vi "Plot Sequence.vi"(5 "Strain Points":dbl[](array[numeric]), 6 "Sliders":T1 {"Instrument Sequence" scale=0.0..1.0; "Strain Sequence" scale=0.0..4.0}, 7 "Instrument Steps":T2, 8 "error in (no error)":errorcluster, 9 "Refnums":T10, 10 "Measurement":T5, 11 "Function":T9) -> (0 "error out":errorcluster)   [LabVIEW 2014]
uses:
  PlotData Refnums.ctl
  Chooseplot.ctl
  Electrical Data Plot Refnums.ctl
  Optical Spectrum Plot Refnum.ctl
  PlotData Functions.ctl
  Measurement.ctl
  WhichInstrument.ctl
  Hardware Control/Parameter Analyzer/Electrical Data.ctl
  Hardware Control/Spectrometer/Spectral Data.ctl
  Instrument Sequence/Instrument Steps.ctl
  Instrument Sequence/Action.ctl
  Instrument Sequence/Instrument List.ctl
panel:
  out "Configuration":string
  out "Measurement Sequence":cluster{"Instrument Sequence":T5[]}[](array[cluster])
  # "LICENSED MATERIALS – PROPERTY OF IBM\nCopyright IBM Corp. 2016,\nALL RIGHTS RESERVED"
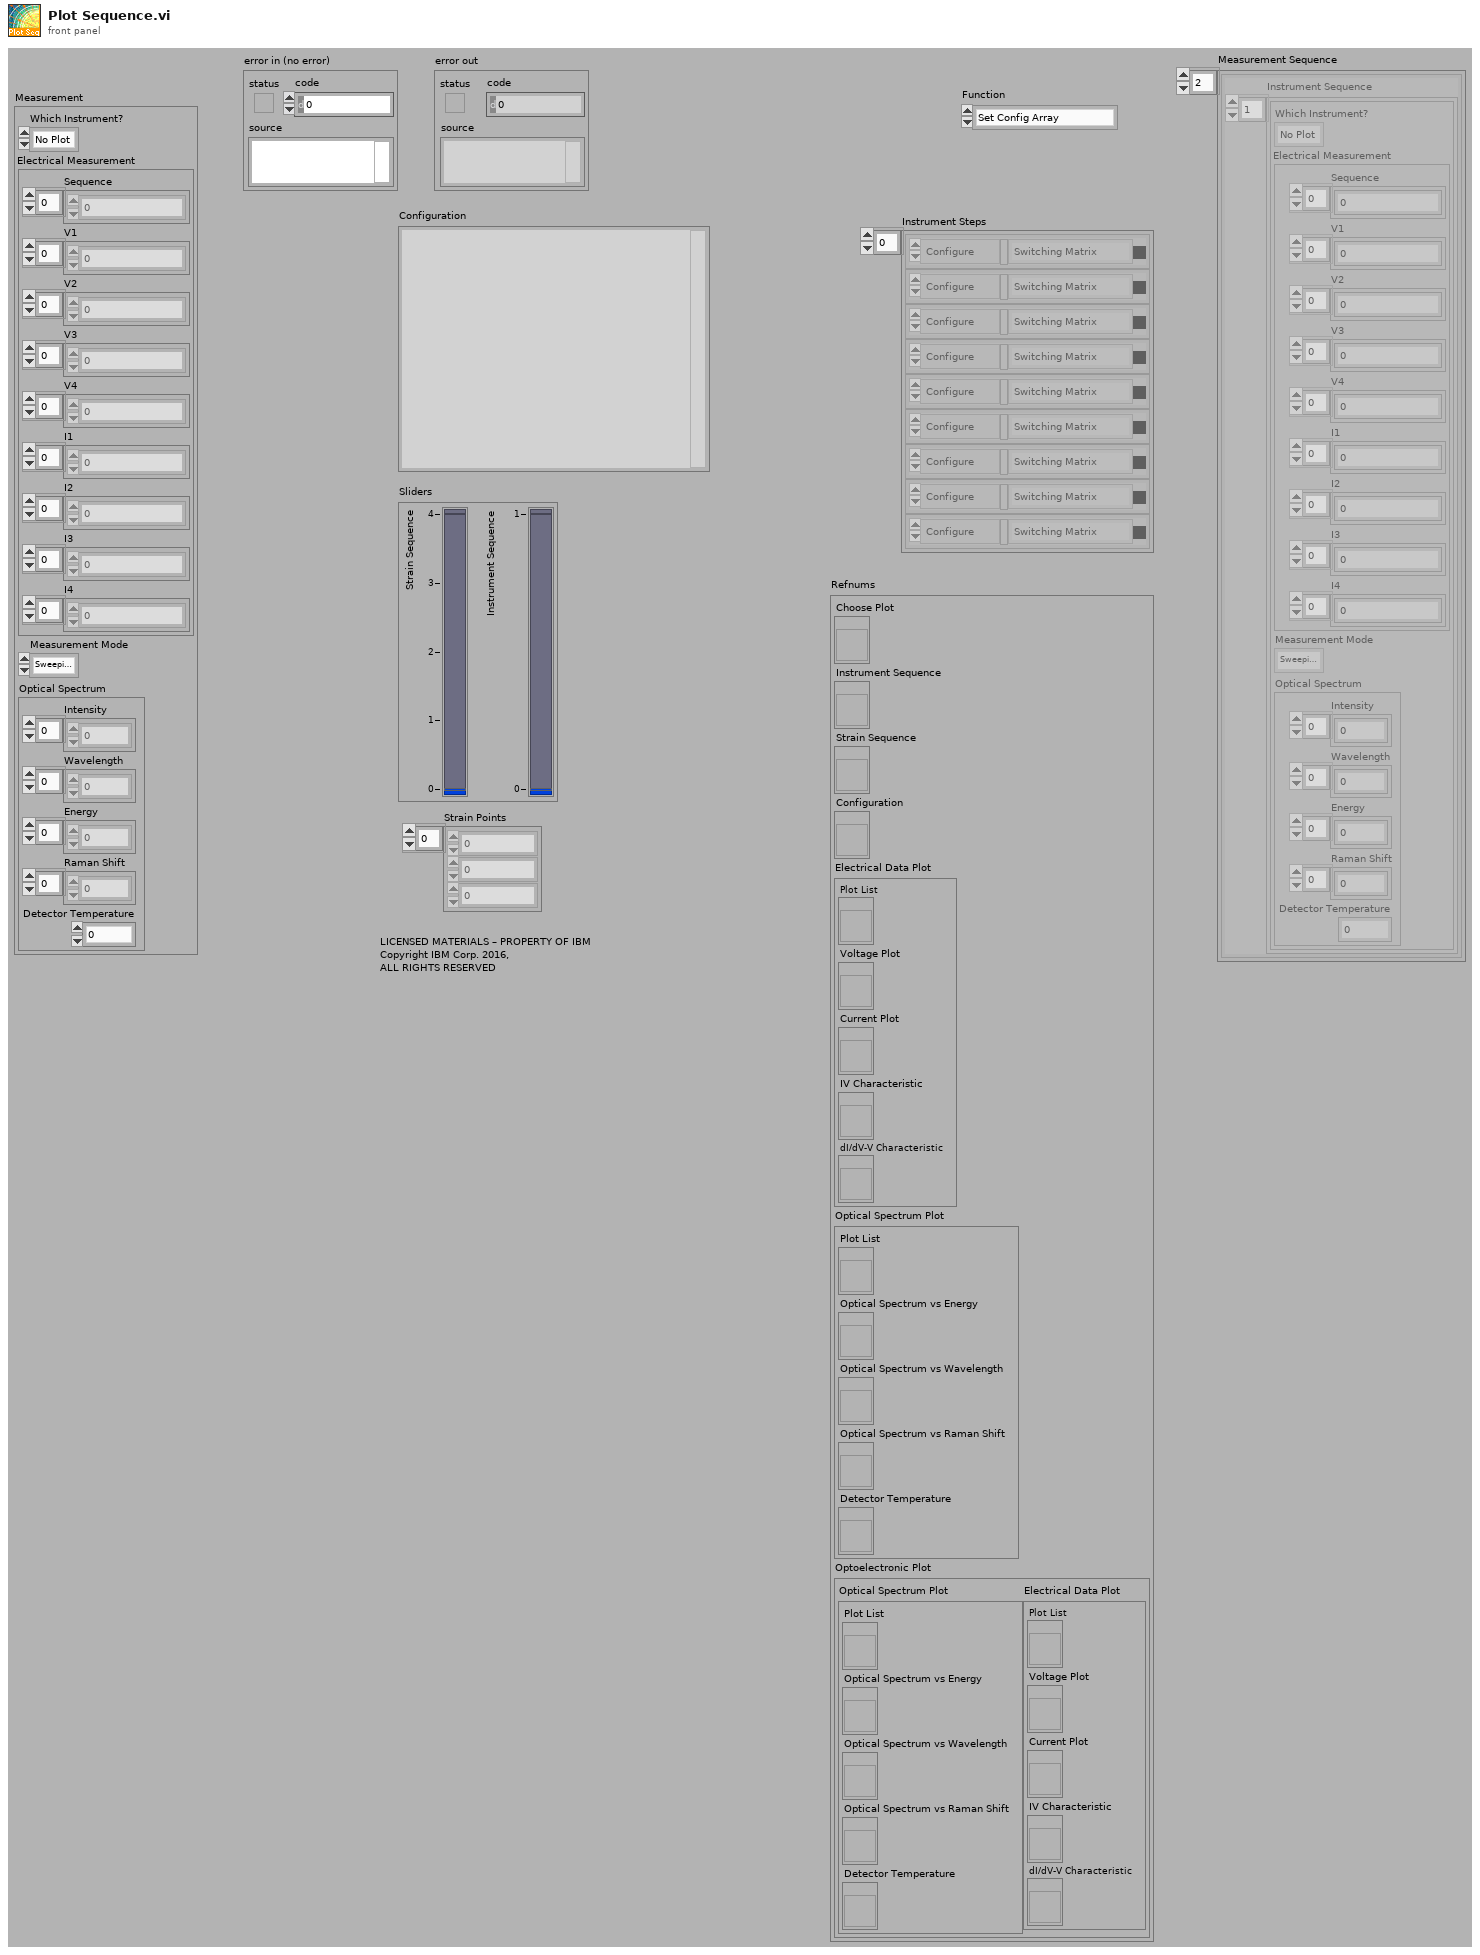
[diagram p1: front panel]
types:
  T1 = cluster{"Strain Sequence":i32, "Instrument Sequence":i32}
  T2 = typedef "Instrument Steps.ctl" = cluster{"Action":T3, "Configuration":variant, "Instrument":T4, "Status":enum8{"False", "True", "Mixed"}}[]
  T3 = typedef "Action.ctl" = enum32{"Configure", "Measure"}
  T4 = typedef "Instrument List.ctl" = enum32{"Unknown Instrument", "Switching Matrix", "Parameter Analyzer", "Optical Spectrometer", "Optoelectronic", "Autofocus"}
  T5 = typedef "Measurement.ctl" = cluster{"Which Instrument?":T6, "Electrical Measurement":T7, "Measurement Mode":enum16{"Sweeping Mode", "Sampling Mode"}, "Optical Spectrum":T8}
  T6 = typedef "WhichInstrument.ctl" = enum16{"No Plot", "Spectrometer", "Parameter Analyzer", "Optoelectronic"}
  T7 = typedef "Electrical Data.ctl" = cluster{"Sequence":dbl[], "V1":dbl[], "V2":dbl[], "V3":dbl[], "V4":dbl[], "I1":dbl[], "I2":dbl[], "I3":dbl[], "I4":dbl[]}
  T8 = typedef "Spectral Data.ctl" = cluster{"Intensity":dbl[], "Wavelength":dbl[], "Energy":dbl[], "Raman Shift":dbl[], "Detector Temperature":dbl}
  T9 = typedef "PlotData Functions.ctl" = enum16{"Set Config Array", "Set Strain Seq. Slider", "Desable Strain Seq. Slider", "Set Instrument Seq. Slider", "Desable Instrument Seq. Slider", "Clear Sequence", "Plot Data", "Append Measurement", "Next Strain Step", "Update Refnums"}
  T10 = typedef "PlotData Refnums.ctl" = cluster{"Choose Plot":refnum<vi>, "Instrument Sequence":refnum<vi>, "Strain Sequence":refnum<vi>, "Configuration":refnum<vi>, "Electrical Data Plot":T11, "Optical Spectrum Plot":T12, "Optoelectronic Plot":cluster{"Optical Spectrum Plot":T12, "Electrical Data Plot":T11}}
  T11 = typedef "Electrical Data Plot Refnums.ctl" = cluster{"Plot List":refnum<vi>, "Voltage Plot":refnum<vi>, "Current Plot":refnum<vi>, "IV Characteristic":refnum<vi>, "dI/dV-V Characteristic":refnum<vi>}
  T12 = typedef "Optical Spectrum Plot Refnum.ctl" = cluster{"Plot List":refnum<vi>, "Optical Spectrum vs Energy":refnum<vi>, "Optical Spectrum vs Wavelength":refnum<vi>, "Optical Spectrum vs Raman Shift":refnum<vi>, "Detector Temperature":refnum<vi>}
  T13 = cluster{"Instrument Sequence":i32, "Measurement Sequence":i32}
  T14 = typedef "SaveData Instrument Configuration.ctl" = cluster{"Instrument":T4, "Configuration":string}
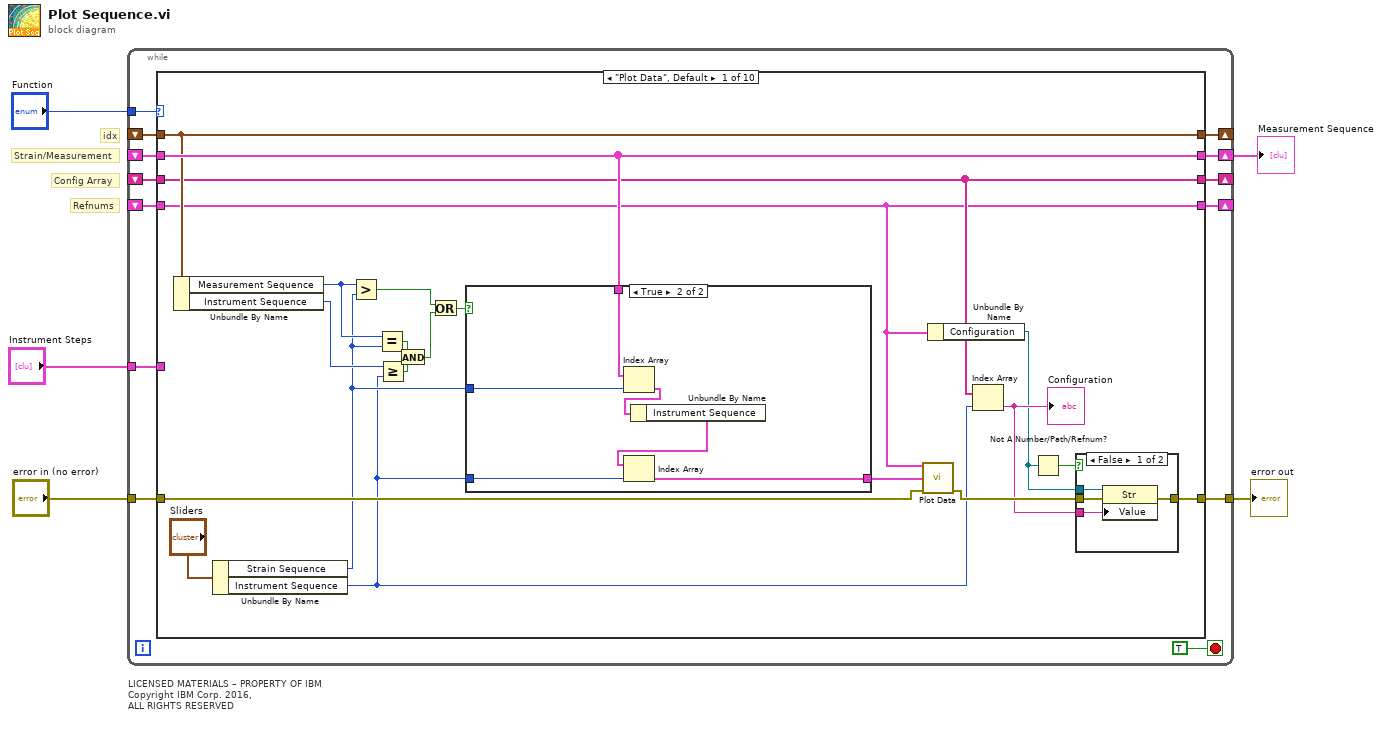
[diagram p0: block diagram]
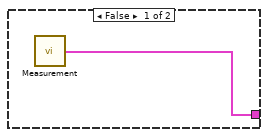
[diagram p3: hidden frame]
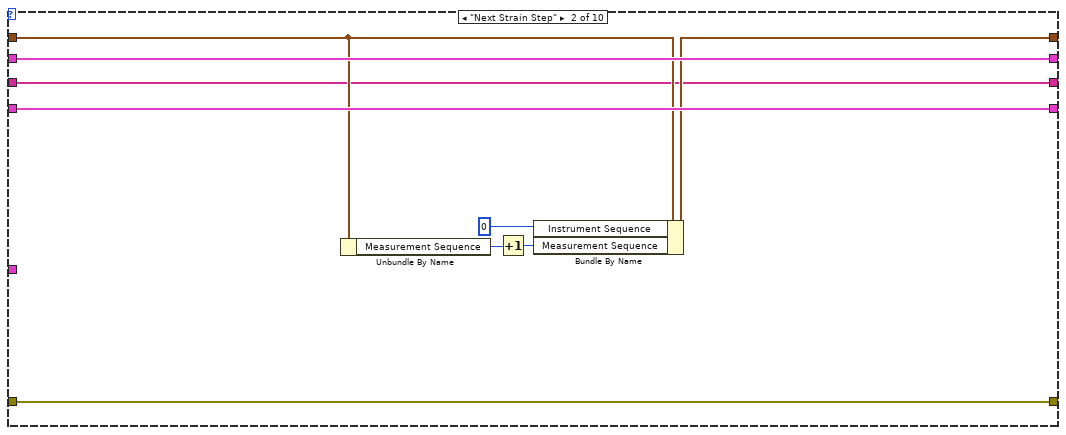
[diagram p4: hidden frame]
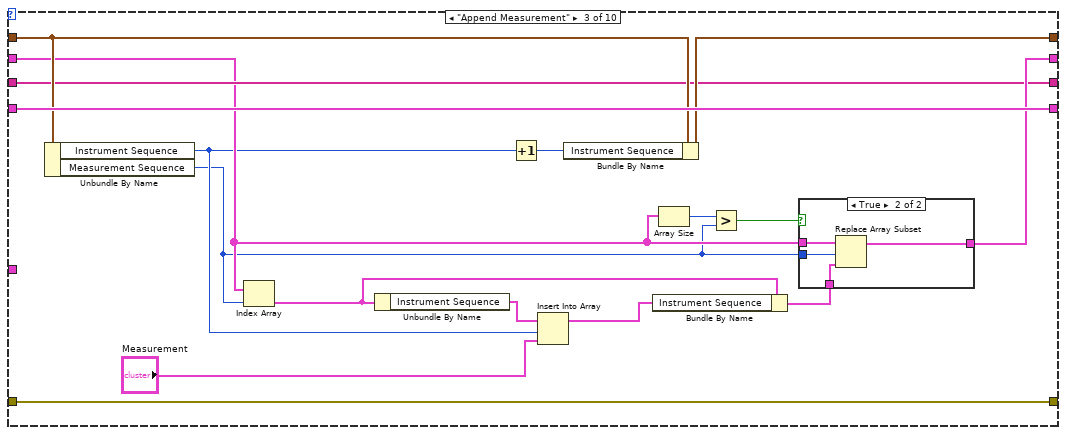
[diagram p5: hidden frame]
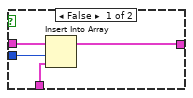
[diagram p6: hidden frame]
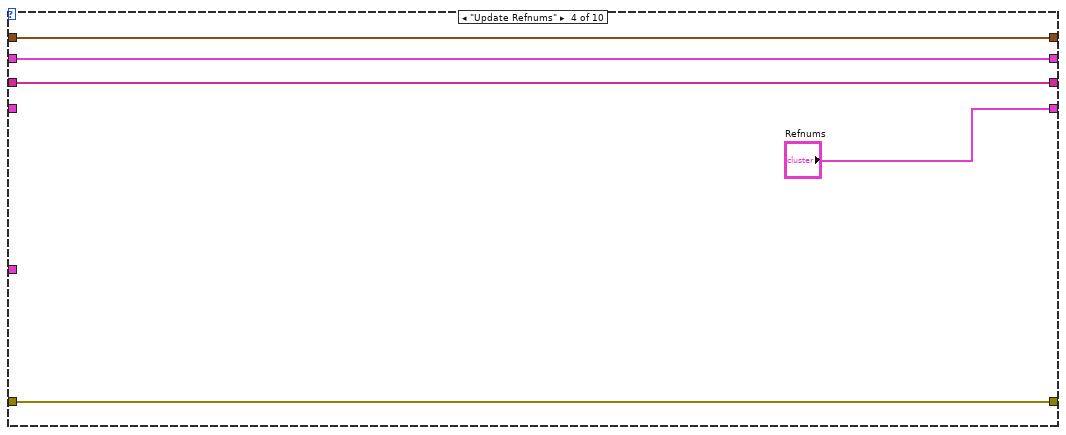
[diagram p7: hidden frame]
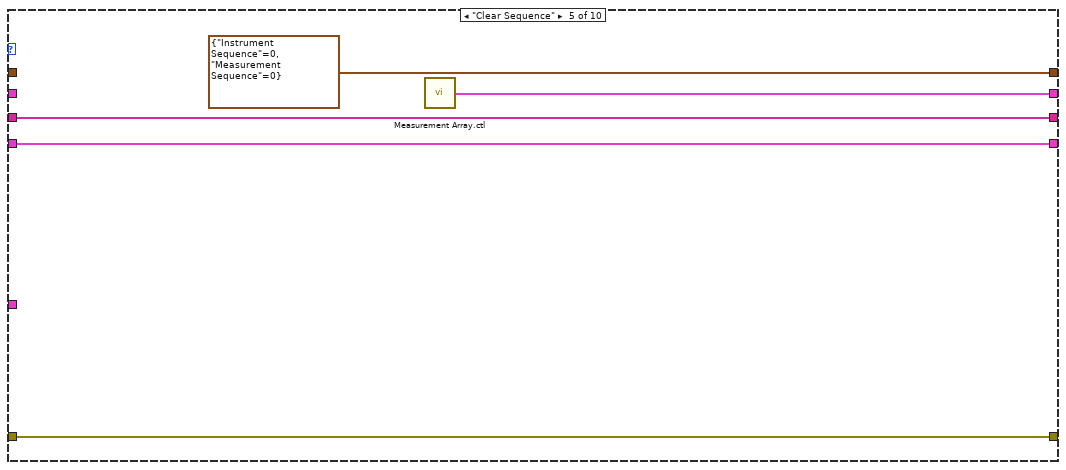
[diagram p8: hidden frame]
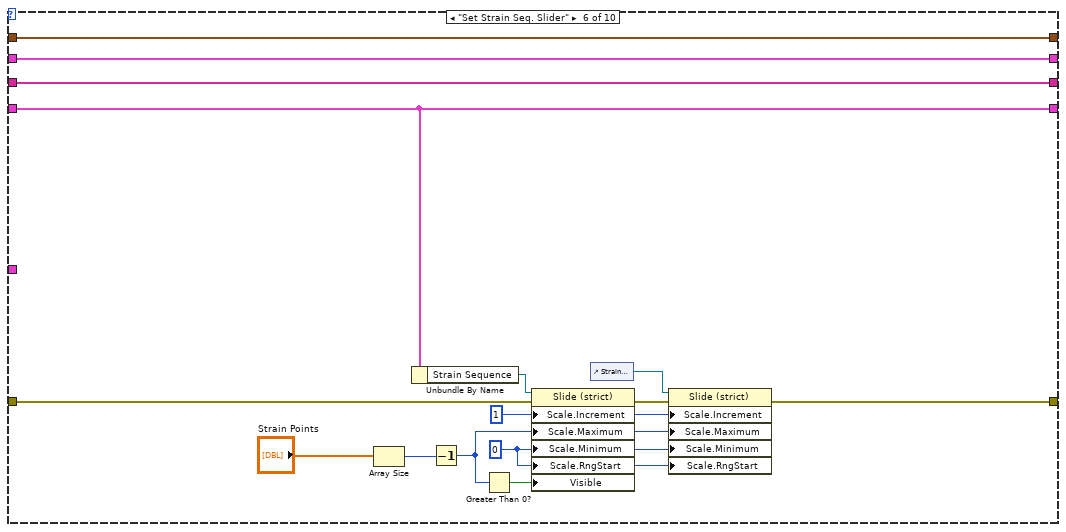
[diagram p9: hidden frame]
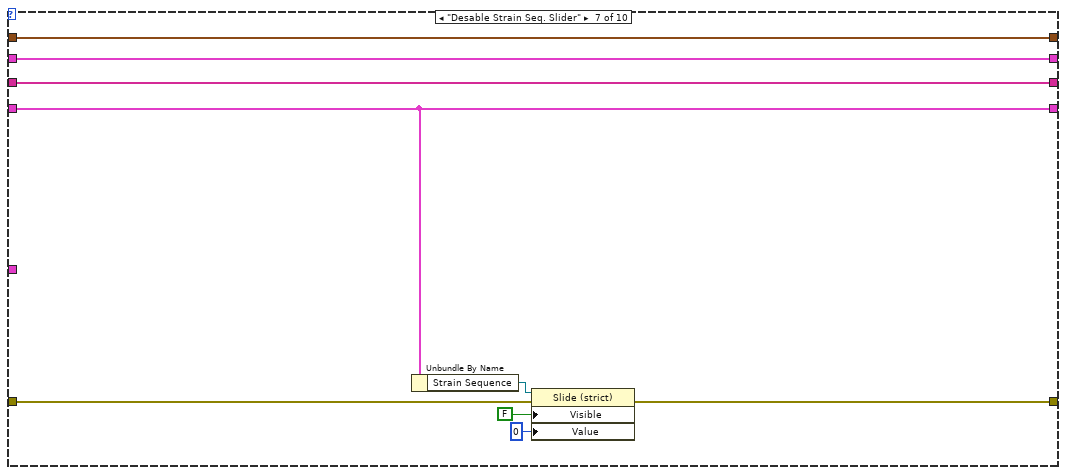
[diagram p10: hidden frame]
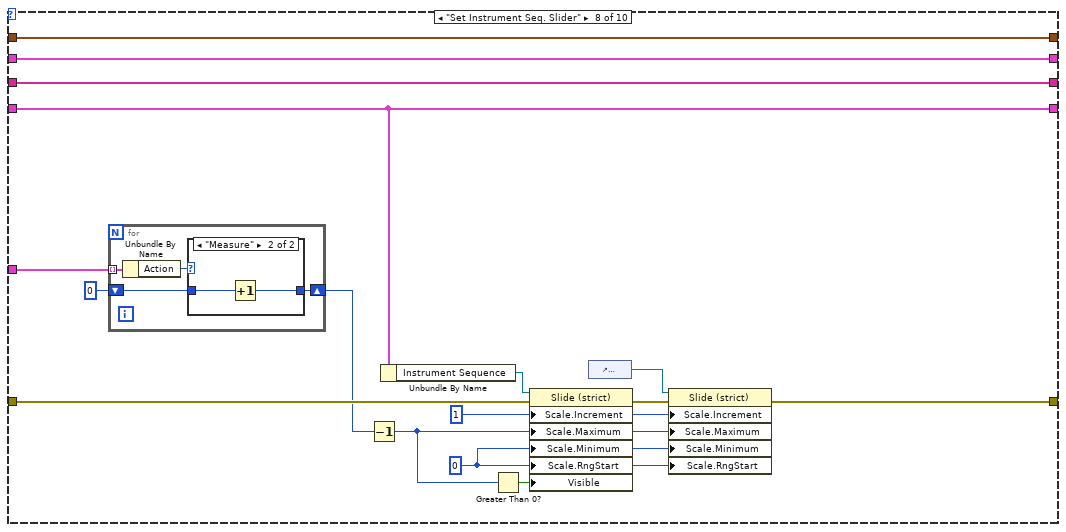
[diagram p11: hidden frame]
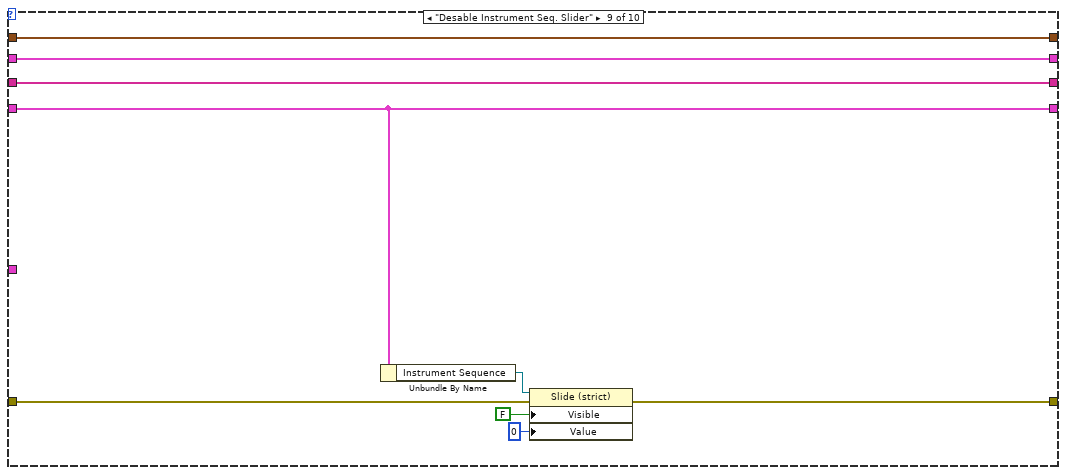
[diagram p13: hidden frame]
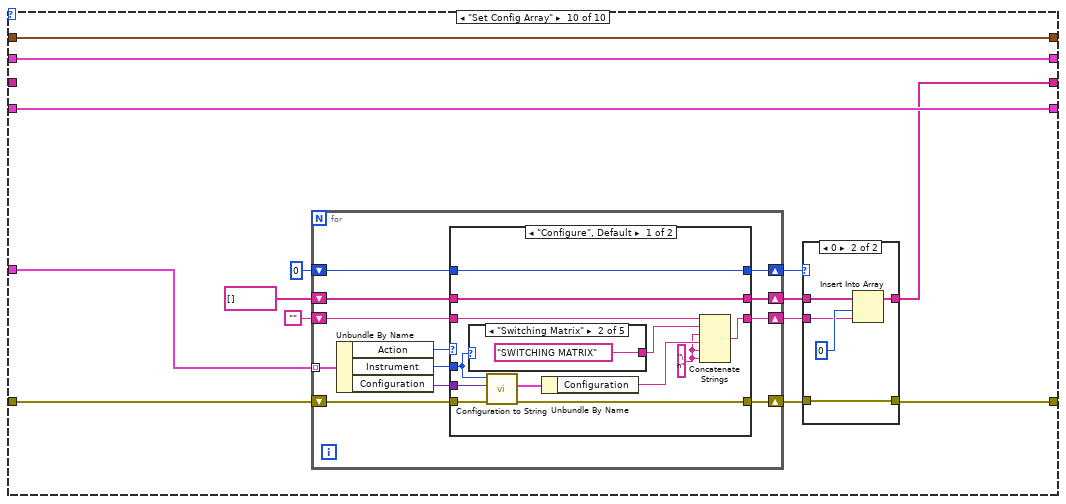
[diagram p14: hidden frame]
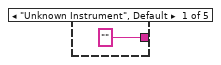
[diagram p16: hidden frame]
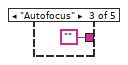
[diagram p17: hidden frame]
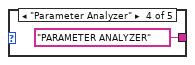
[diagram p18: hidden frame]
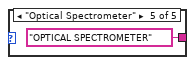
[diagram p19: hidden frame]
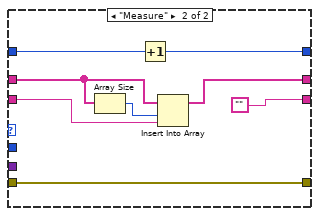
[diagram p20: hidden frame]
diagram:
  # "LICENSED MATERIALS – PROPERTY OF IBM\nCopyright IBM Corp. 2016,\nALL RIGHTS RESERVED"
  # "Config Array"
  # "idx"
  # "Refnums"
  # "Strain/Measurement"
  n1 = while {
    tunnel: "error in (no error)" -> [w18]
    tunnel: [w17] -> w4
    tunnel: "Function" -> [w14]
    shift-right: [w13] -> _
    shift-left: _ -> [w16]
    shift-right: [w12] -> w1
    shift-left: _ -> [w11]
    shift-right: [w10] -> _
    shift-left: _ -> [w9]
    tunnel: "Instrument Steps" -> [w8]
    shift-right: [w7] -> _
    shift-left: _ -> [w6]
    stop <- TRUE stop-if-true
    n2 = case shown="\"Plot Data\", Default" w14 {
      tunnel: w18 -> [w39 w59 w76 w90 w95 w106 w115 w130 w147 w162]
      tunnel: [w26 w59 w76 w90 w95 w100 w113 w124 w145 w156] -> w17
      tunnel: w16 -> [w25 w60 w77 _ w94 w108 w117 w132 w149 w158]
      tunnel: [w25 w60 w77 "Refnums" w94 w108 w117 w132 w149 w158] -> w13
      tunnel: [w37 w58 w72 w88 w91 w109 w118 w133 w150 w160] -> w12
      tunnel: w11 -> [w37 w58 w68 w88 _ w109 w118 w133 w150 w160]
      tunnel: [w35 w57 w75 w87 T13 {"Instrument Sequence"=0, "Measurement Sequence"=0} ("Sequence Index") w110 w119 w134 w151 w161] -> w10
      tunnel: w9 -> [w35 w56 w74 w87 _ w110 w119 w134 w151 w161]
      tunnel: w8 -> [_ _ _ _ _ _ _ w120 _ w163]
      tunnel: [w27 w52 w71 w86 w92 w101 w114 w125 w146 w153] -> w7
      tunnel: w6 -> [w27 w52 w71 w86 w92 w101 w114 w125 w146 _]
      frame "Plot Data", Default {
        n3 = Unbundle By Name(w35) -> ("Measurement Sequence"=w34:i32, "Instrument Sequence"=w33:i32)
        n4 = Unbundle By Name("Sliders") -> ("Strain Sequence"=w20:i32, "Instrument Sequence"=w19:i32)
        n5 = Greater?(x=w34, y=w20) -> (0:w30:bool)
        n6 = Equal?(x=w34, y=w20) -> (x = y?=w32:bool)
        n7 = Greater Or Equal?(x=w33, y=w19) -> (x >= y?=w31:bool)
        n8 = And(x=w32, y=w31) -> (x .and. y?=w29:bool)
        n9 = Or(x=w30, y=w29) -> (x .or. y?=w28:bool)
        n10 = case shown="True" w28 {
          tunnel: w19 -> [_ w51]
          tunnel: w37 -> [_ w50]
          tunnel: [w45 w46] -> w36
          tunnel: w20 -> [_ w49]
          frame False {
            n11 = call "Measurement.vi"() -> ("Measurement"=w45:T5)
          }
          frame True {
            n12 = Index Array(array=w50, index=w49) -> (element=w48:cluster{"Instrument Sequence":T5[]})
            n13 = Unbundle By Name(w48) -> ("Instrument Sequence"=w47:T5[])
            n14 = Index Array(array=w47, index=w51) -> (element=w46:T5)
          }
        }
        n15 = call "Plot Data.vi"("Plots Refnums"=w25, "Measurement"=w36, "error in (no error)"=w39) -> ("error out"=w38:errorcluster)  [unwired: 5 in, 7 out]
        n16 = Unbundle By Name(w25) -> ("Configuration"=w23:refnum<vi>)
        n17 = Index Array(array=w27, index=w19) -> (element=w24:string)
        "Configuration" <- w24
        n18 = Not A Number/Path/Refnum?(number/path/refnum=w23) -> (NaN/Path/Refnum?=w22:bool)
        n19 = case shown="False" w22 {
          tunnel: w38 -> [w43 w44]
          tunnel: [w42 w44] -> w26
          tunnel: w23 -> [w41 _]
          tunnel: w24 -> [w40 _]
          frame False {
            n20 = property class="Str"(reference=w41, error in=w43, "Value"=w40) -> (error out=w42:errorcluster)  [unwired: 1 out]
          }
          frame True {
          }
        }
      }
      frame "Next Strain Step" {
        n21 = Unbundle By Name(w56) -> ("Measurement Sequence"=w54:i32)
        n22 = Increment(x=w54) -> (x+1=w55:i32)
        n23 = Bundle By Name(cluster=w56, "Instrument Sequence"=0, "Measurement Sequence"=w55) -> (w57:T13)
      }
      frame "Append Measurement" {
        n24 = Unbundle By Name(w74) -> ("Instrument Sequence"=w67:i32, "Measurement Sequence"=w63:i32)
        n25 = Index Array(array=w68, index=w63) -> (element=w69:cluster{"Instrument Sequence":T5[]})
        n26 = Unbundle By Name(w69) -> ("Instrument Sequence"=w62:T5[])
        n27 = Increment(x=w67) -> (x+1=w73:i32)
        n28 = Insert Into Array "Insert Into Array"(array=w62, index=w67, new element="Measurement") -> (w65:T5[])
        n29 = Bundle By Name(cluster=w74, "Instrument Sequence"=w73) -> (w75:T13)
        n30 = Bundle By Name(cluster=w69, "Instrument Sequence"=w65) -> (w70:cluster{"Instrument Sequence":T5[]})
        n31 = Array Size(array=w68) -> (size(s)=w61:i32)
        n32 = Greater?(x=w61, y=w63) -> (0:w64:bool)
        n33 = case shown="True" w64 {
          tunnel: w63 -> [w81 w85]
          tunnel: w68 -> [w80 w84]
          tunnel: [w78 w83] -> w72
          tunnel: w70 -> [w79 w82]
          frame False {
            n34 = Insert Into Array "Insert Into Array"(array=w80, index=w81, new element=w79) -> (w78:cluster{"Instrument Sequence":T5[]}[])
          }
          frame True {
            n35 = Replace Array Subset "Replace Array Subset"(array=w84, new element=w82, index=w85) -> (w83:cluster{"Instrument Sequence":T5[]}[])
          }
        }
      }
      frame "Update Refnums" {
      }
      frame "Clear Sequence" {
        n36 = call "Measurement Array.ctl"() -> ("Measurement Sequence"=w91:cluster{"Instrument Sequence":T5[]}[])  [unwired: 1 out]
      }
      frame "Set Strain Seq. Slider" {
        w102 = 0
        w103 = 1
        n37 = Array Size(array="Strain Points") -> (size(s)=w98:i32)
        n38 = Unbundle By Name(w108) -> ("Strain Sequence"=w107:refnum<vi>)
        n39 = Decrement(x=w98) -> (x-1=w97:i32)
        n40 = Greater Than 0?(x=w97) -> (x > 0?=w99:bool)
        n41 = property class="Slide (strict)"(reference=w107, error in=w106, "Scale.Increment"=w103, "Scale.Maximum"=w97, "Scale.Minimum"=w102, "Scale.RngStart"=w102, "Visible"=w99) -> (error out=w105:errorcluster)  [unwired: 1 out]
        n42 = control-ref of="Strain Sequence"() -> (w104:refnum<vi>)
        n43 = property class="Slide (strict)"(reference=w104, error in=w105, "Scale.Increment"=w103, "Scale.Maximum"=w97, "Scale.Minimum"=w102, "Scale.RngStart"=w102) -> (error out=w100:errorcluster)  [unwired: 1 out]
      }
      frame "Desable Strain Seq. Slider" {
        n44 = Unbundle By Name(w117) -> ("Strain Sequence"=w116:refnum<vi>)
        n45 = property class="Slide (strict)"(reference=w116, error in=w115, "Visible"=FALSE, "Value"=0) -> (error out=w113:errorcluster)  [unwired: 1 out]
      }
      frame "Set Instrument Seq. Slider" {
        w126 = 0
        w127 = 1
        n46 = for {
          tunnel: w120 -> [w139] mode=indexing
          shift-right: [w136] -> w122
          shift-left: 0 -> [w137]
          n47 = Unbundle By Name(w139) -> ("Action"=w138:T3)
          n48 = case shown="\"Measure\"" w138 {
            tunnel: w137 -> [w140 w141]
            tunnel: [w140 w142] -> w136
            frame "Configure", Default {
            }
            frame "Measure" {
              n49 = Increment(x=w141) -> (x+1=w142:i32)
            }
          }
        }
        n50 = Decrement(x=w122) -> (x-1=w121:i32)
        n51 = Unbundle By Name(w132) -> ("Instrument Sequence"=w131:refnum<vi>)
        n52 = Greater Than 0?(x=w121) -> (x > 0?=w123:bool)
        n53 = property class="Slide (strict)"(reference=w131, error in=w130, "Scale.Increment"=w127, "Scale.Maximum"=w121, "Scale.Minimum"=w126, "Scale.RngStart"=w126, "Visible"=w123) -> (error out=w129:errorcluster)  [unwired: 1 out]
        n54 = control-ref of="Instrument Sequence"() -> (w128:refnum<vi>)
        n55 = property class="Slide (strict)"(reference=w128, error in=w129, "Scale.Increment"=w127, "Scale.Maximum"=w121, "Scale.Minimum"=w126, "Scale.RngStart"=w126) -> (error out=w124:errorcluster)  [unwired: 1 out]
      }
      frame "Desable Instrument Seq. Slider" {
        n56 = Unbundle By Name(w149) -> ("Instrument Sequence"=w148:refnum<vi>)
        n57 = property class="Slide (strict)"(reference=w148, error in=w147, "Visible"=FALSE, "Value"=0) -> (error out=w145:errorcluster)  [unwired: 1 out]
      }
      frame "Set Config Array" {
        n58 = for {
          tunnel: w163 -> [w184] mode=indexing
          shift-right: [w181] -> w157
          shift-left: w162 -> [w182]
          shift-right: [w175] -> w154
          shift-left: string[] [] -> [w176]
          shift-right: [w178] -> w152
          shift-left: "" -> [w179]
          shift-right: [w174] -> w155
          shift-left: 0 -> [w173]
          n59 = Unbundle By Name(w184) -> ("Action"=w177:T3, "Instrument"=w180:T4, "Configuration"=w183:variant)
          n60 = case shown="\"Configure\", Default" w177 {
            tunnel: w183 -> [w196 _]
            tunnel: w182 -> [w195 w209]
            tunnel: [w194 w209] -> w181
            tunnel: w180 -> [w187 _]
            tunnel: w179 -> [w193 w207]
            tunnel: [w191 ""] -> w178
            tunnel: w176 -> [w190 w205]
            tunnel: [w190 w204] -> w175
            tunnel: [w189 w202] -> w174
            tunnel: w173 -> [w189 w203]
            frame "Configure", Default {
              w185 = "\n" ("string")
              n61 = case shown="\"Switching Matrix\"" w187 {
                tunnel: ["" "SWITCHING MATRIX" "" "PARAMETER ANALYZER" "OPTICAL SPECTROMETER"] -> w186
                frame "Unknown Instrument", Default {
                }
                frame "Switching Matrix" {
                }
                frame "Autofocus" {
                }
                frame "Parameter Analyzer" {
                }
                frame "Optical Spectrometer" {
                }
              }
              n62 = call "Configuration to String.vi"("error in (no error)"=w195, "Configuration"=w196, "Instrument"=w187) -> ("error out"=w194:errorcluster, "Instrument Configuration"=w192:T14)  [unwired: 7 out]
              n63 = Unbundle By Name(w192) -> ("Configuration"=w188:string)
              n64 = Concatenate Strings(w193, w186, w185, w188, w185, w185) -> (w191:string)
            }
            frame "Measure" {
              n65 = Array Size(array=w205) -> (size(s)=w206:i32)
              n66 = Increment(x=w203) -> (x+1=w202:i32)
              n67 = Insert Into Array(array=w205, index=w206, new element=w207) -> (w204:string[])
            }
          }
        }
        n68 = case shown="0" w155 {
          tunnel: w157 -> [w167 w172]
          tunnel: [w167 w172] -> w156
          tunnel: w154 -> [w166 w170]
          tunnel: [w166 w171] -> w153
          tunnel: w152 -> [_ w168]
          frame Default {
          }
          frame 0 {
            n69 = Insert Into Array(array=w170, index=0, new element=w168) -> (w171:string[])
          }
        }
      }
    }
  }
  "error out" <- w4
  "Measurement Sequence" <- w1
